vi "Wait notifier.vi"(8 "error in (no error)":errorcluster caption="entrée d'erreur (pas d'erreur)", 9 "ignorer les précédents (F)":bool, 10 "timeout in ms (-1)":i32=-1, 11 "Message en entrée":refnum<class "Message.lvclass">) -> (0 "error out":errorcluster caption="sortie d'erreur", 2 "notification":variant, 3 "Message en sortie":refnum<class "Message.lvclass">)   [LabVIEW 2015, in "Message.lvclass"]
uses:
  Message.lvclass
  Message.lvclass/Message.ctl
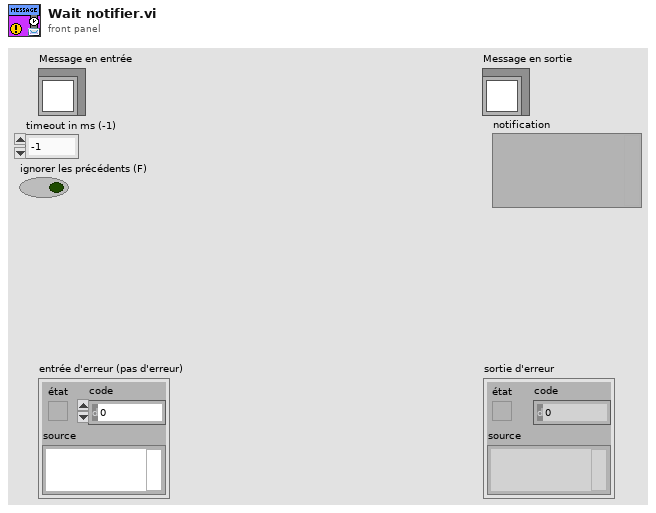
[diagram p1: front panel]
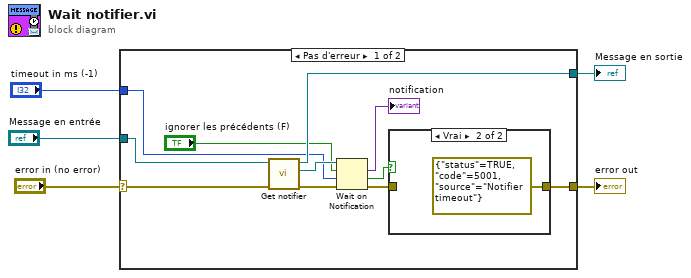
[diagram p0: block diagram]
diagram:
  n1 = case shown="Pas d'erreur" "error in (no error)" {
    selector: "error in (no error)" -> [w14 w20]
    tunnel: [w9 w20] -> w4
    tunnel: [w12 w19] -> w2
    tunnel: "Message en entrée" -> [w15 w19]
    tunnel: "timeout in ms (-1)" -> [w11 _]
    frame No Error {
      n2 = call "Get notifier.vi"("error in (no error)"=w14, "Message en entrée"=w15) -> ("error out"=w13:errorcluster, "notifier"=w16:refnum<notifier>, "Message en sortie"=w12:refnum<class "Message.lvclass">)  [unwired: 7 in]
      n3 = Wait on Notification(notifier=w16, ignore previous (F)="ignorer les précédents (F)", timeout in ms (-1)=w11, error in (no error)=w13) -> (notification=→"notification":variant, timed out?=w10:bool, error out=w8:errorcluster)  [unwired: 1 out]
      n4 = case shown="Vrai" w10 {
        tunnel: [w17 errorcluster {"status"=TRUE, "code"=5001, "source"="Notifier timeout"} ("error out")] -> w9
        tunnel: w8 -> [w17 _]
        frame False {
        }
        frame True {
        }
      }
    }
    frame Error {
    }
  }
  "error out" <- w4
  "Message en sortie" <- w2
